vi "Restore Event Data.vi"(8 "error in":errorcluster, 10 "Path":path, 11 "TDMS in":refnum<class "TDMS.lvclass">) -> (0 "error out":errorcluster, 3 "TDMS out":refnum<class "TDMS.lvclass">)   [LabVIEW 2019, in "TDMS.lvlib" / "TDMS.lvclass"]
uses:
  TDMS.lvclass
  TDMS.lvclass/TDMS.ctl
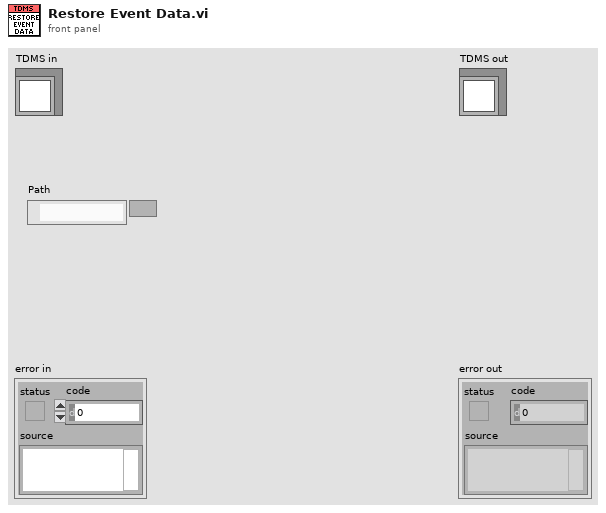
[diagram p1: front panel]
types:
  T1 = cluster{"Time":timestamp[], "Instrument":string[], "Description":string[], "Data":string[]}
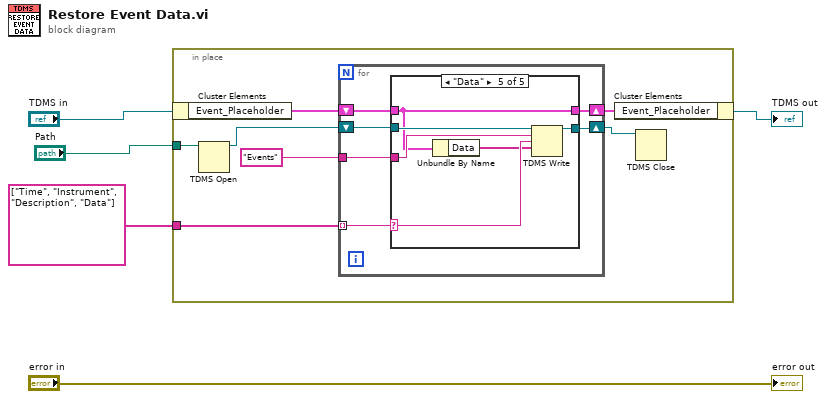
[diagram p0: block diagram]
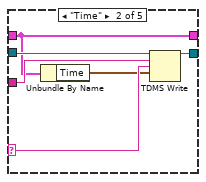
[diagram p3: hidden frame]
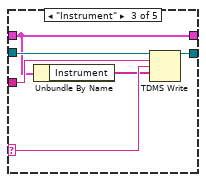
[diagram p4: hidden frame]
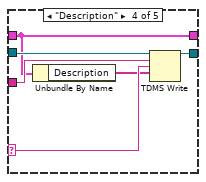
[diagram p5: hidden frame]
diagram:
  n1 = in-place {
    in-place-border: string[] ["Time", "Instrument", "Description", "Data"] -> [w12]
    in-place-border: "Path" -> [w8]
    n2 = in-place-cluster #1("TDMS in") -> ("Event_Placeholder"=w11:T1)
    n3 = TDMS Open(11:w8) -> (3:w7:refnum<k34>)  [unwired: 6 in, 1 out]
    n4 = for {
      tunnel: w12 -> [w18] mode=indexing
      shift-right: [w16] -> w6
      shift-left: w7 -> [w17]
      shift-right: [w13] -> w10
      shift-left: w11 -> [w14]
      tunnel: "Events" -> [w15]
      n5 = case shown="\"Data\"" w18 {
        selector: w18 -> [_ w23 w29 w35 w41]
        tunnel: w17 -> [w19 w26 w32 w38 w44]
        tunnel: [w19 w25 w31 w37 w43] -> w16
        tunnel: w15 -> [_ w24 w30 w36 w42]
        tunnel: w14 -> [w20 w21 w27 w33 w39]
        tunnel: [w20 w21 w27 w33 w39] -> w13
        frame "False", Default {
        }
        frame "Time" {
          n6 = Unbundle By Name(w21) -> ("Time"=w22:timestamp[])
          n7 = TDMS Write(0:w26, 5:w24, 7:w23, 9:w22) -> (4:w25:refnum<k34>)  [unwired: 2 in, 3 out]
        }
        frame "Instrument" {
          n8 = Unbundle By Name(w27) -> ("Instrument"=w28:string[])
          n9 = TDMS Write(0:w32, 5:w30, 7:w29, 9:w28) -> (4:w31:refnum<k34>)  [unwired: 2 in, 3 out]
        }
        frame "Description" {
          n10 = Unbundle By Name(w33) -> ("Description"=w34:string[])
          n11 = TDMS Write(0:w38, 5:w36, 7:w35, 9:w34) -> (4:w37:refnum<k34>)  [unwired: 2 in, 3 out]
        }
        frame "Data" {
          n12 = Unbundle By Name(w39) -> ("Data"=w40:string[])
          n13 = TDMS Write(0:w44, 5:w42, 7:w41, 9:w40) -> (4:w43:refnum<k34>)  [unwired: 2 in, 3 out]
        }
      }
    }
    n14 = in-place-cluster #1("Event_Placeholder"=w10) -> (→"TDMS out":refnum<class "TDMS.lvclass">)
    n15 = TDMS Close(11:w6) -> ()  [unwired: 1 in, 2 out]
  }
  "error out" <- "error in"
